vi "Build Set of Infinite Regions.vi"(11 "Closest Point Indices":i32[][](array[numeric])) -> (3 "Infinite Regions":set{i32}(c389))   [LabVIEW 2019]
doc: "Build a set of all regions that occupy the edges of the Manhattan Distance map."
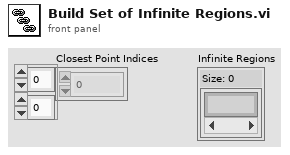
[diagram p1: front panel]
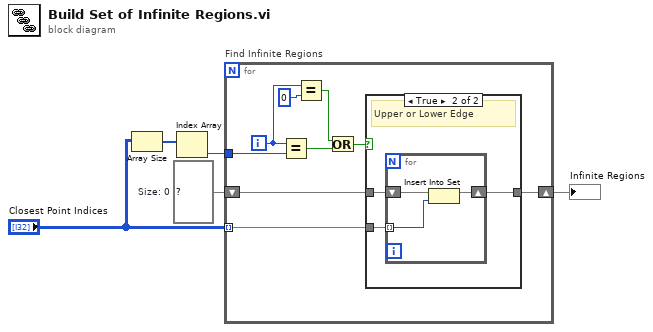
[diagram p0: block diagram]
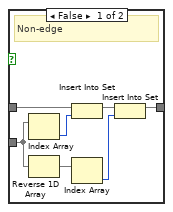
[diagram p2: hidden frame]
diagram:
  w3 = set{i32} {}  # Size: 0
  n1 = Array Size(array="Closest Point Indices") -> (size(s)=w1:i32[])
  n2 = Index Array(array=w1) -> (element=w2:i32)  [unwired: 1 in]
  n3 = for "Find Infinite Regions" {
    tunnel: "Closest Point Indices" -> [w9] mode=indexing
    tunnel: w2 -> [w11]
    shift-right: [w7] -> w5
    shift-left: w3 -> [w8]
    i -> [w12]
    n4 = Equal?(x=w12, y=w11) -> (x = y?=w14:bool)
    n5 = Equal?(x=w12, y=0) -> (x = y?=w13:bool)
    n6 = Or(x=w13, y=w14) -> (x .or. y?=w6:bool)
    n7 = case shown="True" w6 {
      tunnel: w9 -> [w18 w24]
      tunnel: w8 -> [w21 w23]
      tunnel: [w19 w22] -> w7
      frame False {
        # "Non-edge"
        n8 = Index Array(array=w18) -> (element=w16:i32)  [unwired: 1 in]
        n9 = Reverse 1D Array(array=w18) -> (reversed array=w17:i32[])
        n10 = Insert Into Set(10:w16, 11:w21) -> (3:w20:set{i32})  [unwired: 1 out]
        n11 = Index Array(array=w17) -> (element=w15:i32)  [unwired: 1 in]
        n12 = Insert Into Set(10:w15, 11:w20) -> (3:w19:set{i32})  [unwired: 1 out]
      }
      frame True {
        # "Upper or Lower Edge"
        n13 = for {
          tunnel: w24 -> [w25] mode=indexing
          shift-right: [w26] -> w22
          shift-left: w23 -> [w27]
          n14 = Insert Into Set(10:w25, 11:w27) -> (3:w26:set{i32})  [unwired: 1 out]
        }
      }
    }
  }
  "Infinite Regions" <- w5
